vi "gui_T1.vi"(10 "input_xyz":T1) -> ()   [LabVIEW 2018]
uses:
  <vilib>/Analysis/NI_AALBase.lvlib
panel:
  out "particle_lost":bool
  in  "recenter_period_s":u32=5
  in  "recenter":bool=TRUE
  in  "show_all":bool
  in  "hide_all":bool
  out "elapsed_time_HMS":string
  out "estimated_time_HMS":string
  in  "plot_pulses":bool
  in  "gates_calculation":enum16{"Software", "Hardware"}(ring)=enum."Hardware"
  out "pulses":u32[][](graph)
  out "detections":u32[](graph)
  out "std. dev.":dbl format="%.3f"
  out "mean":dbl format="%0.2f"
  in  "auto_normalize":bool
  in  "normalize":bool
  in  "normalization_value":dbl=1.0 caption="Normalization value:" min=1.0 step=1.0
  out "status":string
  in  "use_proposed_width":bool
  in  "calc_width":bool
  in  "start":bool caption="Start"
  in  "save_file":bool
  out "contrast":dbl caption="Contrast :" format="%#_3f"
  in  "show_photons":bool
  in  "show_flags":bool
  out "mse":cluster{"read_widths_us":dbl[], "mse":dbl[]}(graph)
  in  "use_proposed_correction":bool
  out "proposed_read_width_us":dbl
  out "proposed_correction_us":dbl
  out "histogram":cluster{"histogram":i32[], "q_photons":i32[]}(graph)
  out "file_name":string caption="File name :"
  in  "sampling_mode":enum16{"Normal", "Sweep"}(ring)=enum."Sweep"
  out "quality":bool
  out "mse":dbl caption="Mean Square Error" format="%#.2e"
  out "T1_us":dbl format="%#.3g"
  out "T1 curves":cluster{dbl[], "dark_time_us":dbl[]}[](graph)
  in  "correction_us":dbl=0.65 caption="Delay"
  out "stop_count_photon":u32(colorbox)=16776704 caption="Stop Count & photon"
  out "stop_count":u32(colorbox)=6618880 caption="Stop Count"
  out "start_count_photon":u32(colorbox)=14417925 caption="Start Count & photon"
  out "start_count":u32(colorbox)=255 caption="Start Count"
  out "photon":u32(colorbox)=16448250 caption="Photon"
  out "noPhoton":u32(colorbox) caption="No Photon"
  out "photons_chart":u32[][](graph)
  in  "load_file":bool
  in  "refit":bool
  in  "read_width_us":dbl=1.0 caption="Width" min=0.0 max=10000.0 format="%#.3f"
  in  "read_delay_us":dbl caption="Delay"
  out "min_step":dbl format="%#.3f"
  in  "q_samples":i32=50
  in  "dt_stop_us":dbl=10000.0
  in  "dt_start_us":dbl=0.2
  in  "stop":bool
  in  "repetitions":i32=10000 caption="Repetitions" min=1 step=1
  in  "pulse_width_us":dbl=5.0 caption="Pulse width"
  # "Dark time [us]"
  # "*"
  # "*"
  # "us"
  # "*read_width_us and correction_us have to be multiple of 10ns\n*** start and stop markers are inside the detection gate. [start, stop]"
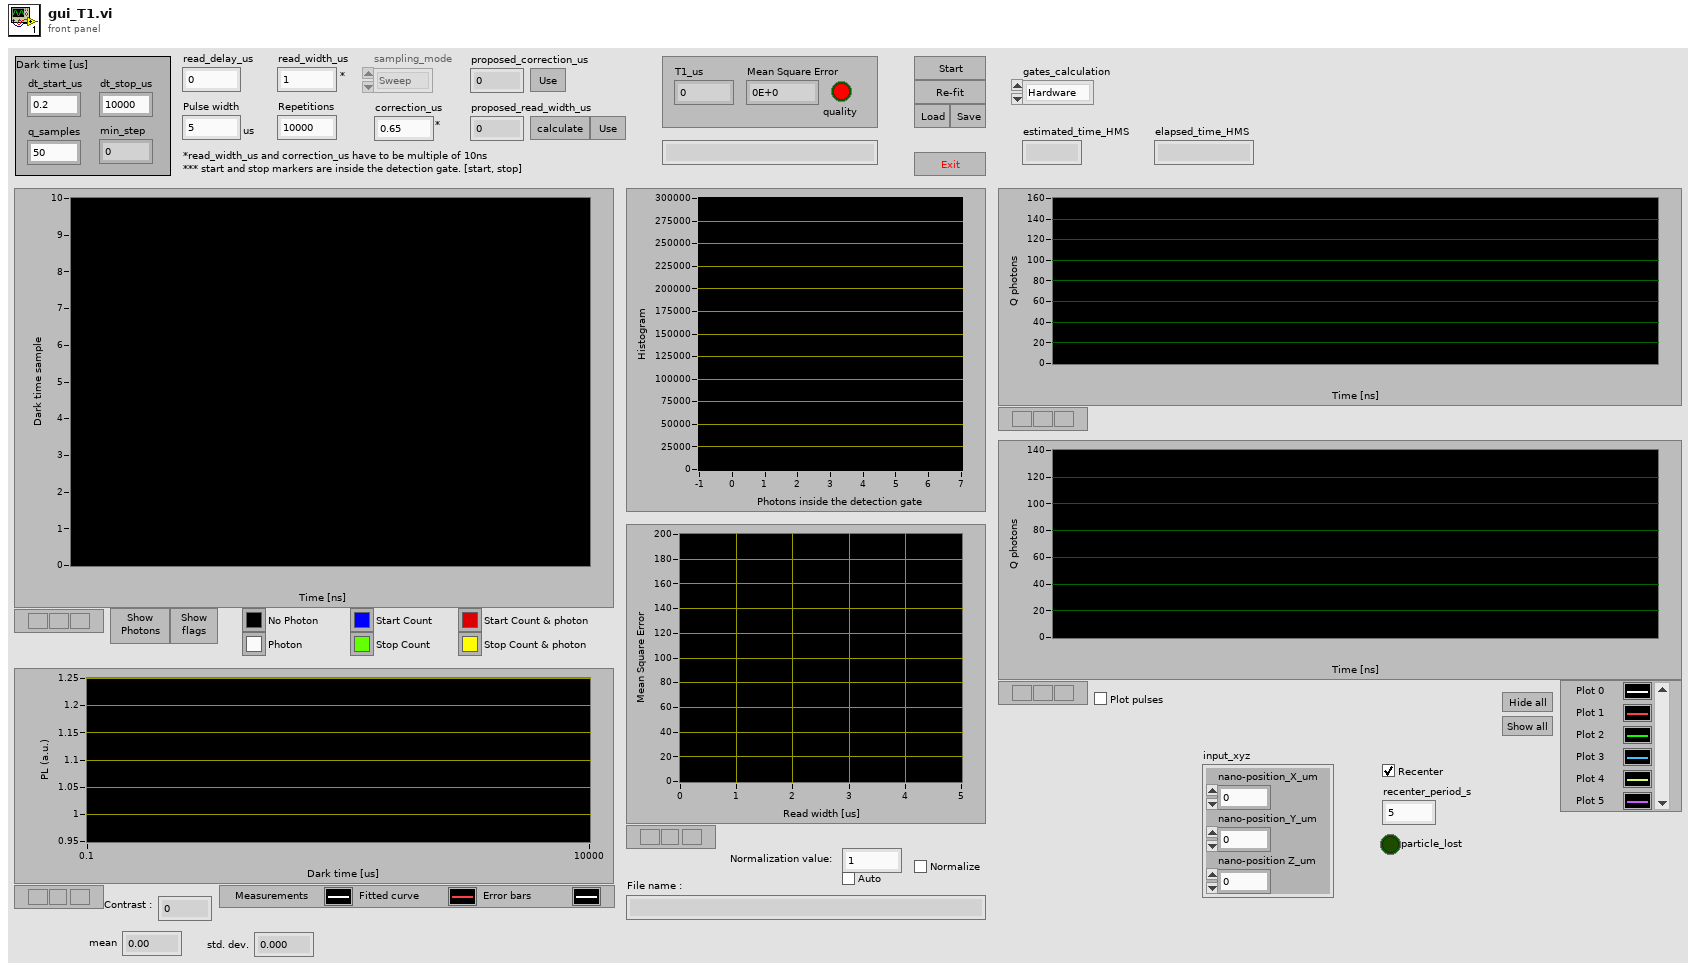
[diagram p1: front panel]
types:
  T1 = cluster{"nano-position_X_um":sgl, "nano-position_Y_um":sgl, "nano-position Z_um":sgl}
  T2 = cluster{"file_path":path, "file_name":string, "image":dbl[][][], "image_size_xy":cluster{"image_size_x_um":sgl, "image_size_y_um":sgl}, "pixel_dwell_time_ms":sgl, "Laser_power_mW":sgl, "pixel_size":dbl, "tile_ij":cluster{"tile_i":i32, "tile_j":i32}, "Objective":string, "ColorMarkers":cluster{dbl, u32}[], "timestamp":timestamp, "micro-position-xyz":cluster{"micro-position_x_mm":sgl, "micro-position_y_mm":sgl, "micro-position_z_mm":sgl}, "zero_xyz":cluster{"zero_x_mm":dbl, "zero_y_mm":dbl, "zero_z_mm":dbl}, "nano-position-xyz":cluster{"nano-position_x_V":sgl, "nano-position_y_V":sgl, "nano-position_z_V":sgl}, "Kxyz":cluster{"Kx_V/um":sgl, "Ky_V/um":sgl, "Kz_V/um":sgl}}
  T3 = cluster{"x_um":sgl[], "y_um":sgl[], "z_um":sgl[], "timetag":timestamp[]}
  T4 = cluster{"sampling_times":dbl[], "fitted_signal":dbl[]}
  T5 = cluster{"Ie":dbl, "Cm":dbl, "Tm":dbl, "C1":dbl, "T1":dbl, "mse":dbl}
  T6 = cluster{"dark_times_us":dbl[], "pulse_width_us":dbl, "read_delay_us":dbl, "read_width_us":dbl, "repetitions":i32, "sampling_mode":enum16{"Normal", "Sweep"}, "correction_us":dbl}
  T7 = cluster{"input_xyz":cluster{"nano-position_X_um":sgl, "nano-position_Y_um":sgl, "nano-position Z_um":sgl}, "recenter":bool, "recenter_s":u32}
  T8 = enum16{"standby", "doT1", "abort", "save", "re-fit", "load", "refresh", "use_proposed", "calcWidth"}
  T9 = cluster{"Ie":dbl, "A":dbl, "Ta":dbl, "B":dbl, "Tb":dbl, "mse":dbl}
  T10 = cluster{"dark_times":dbl[], "fitted_signal":dbl[]}
  T11 = cluster{"dark_times_us":dbl[], "measured_signal":dbl[]}
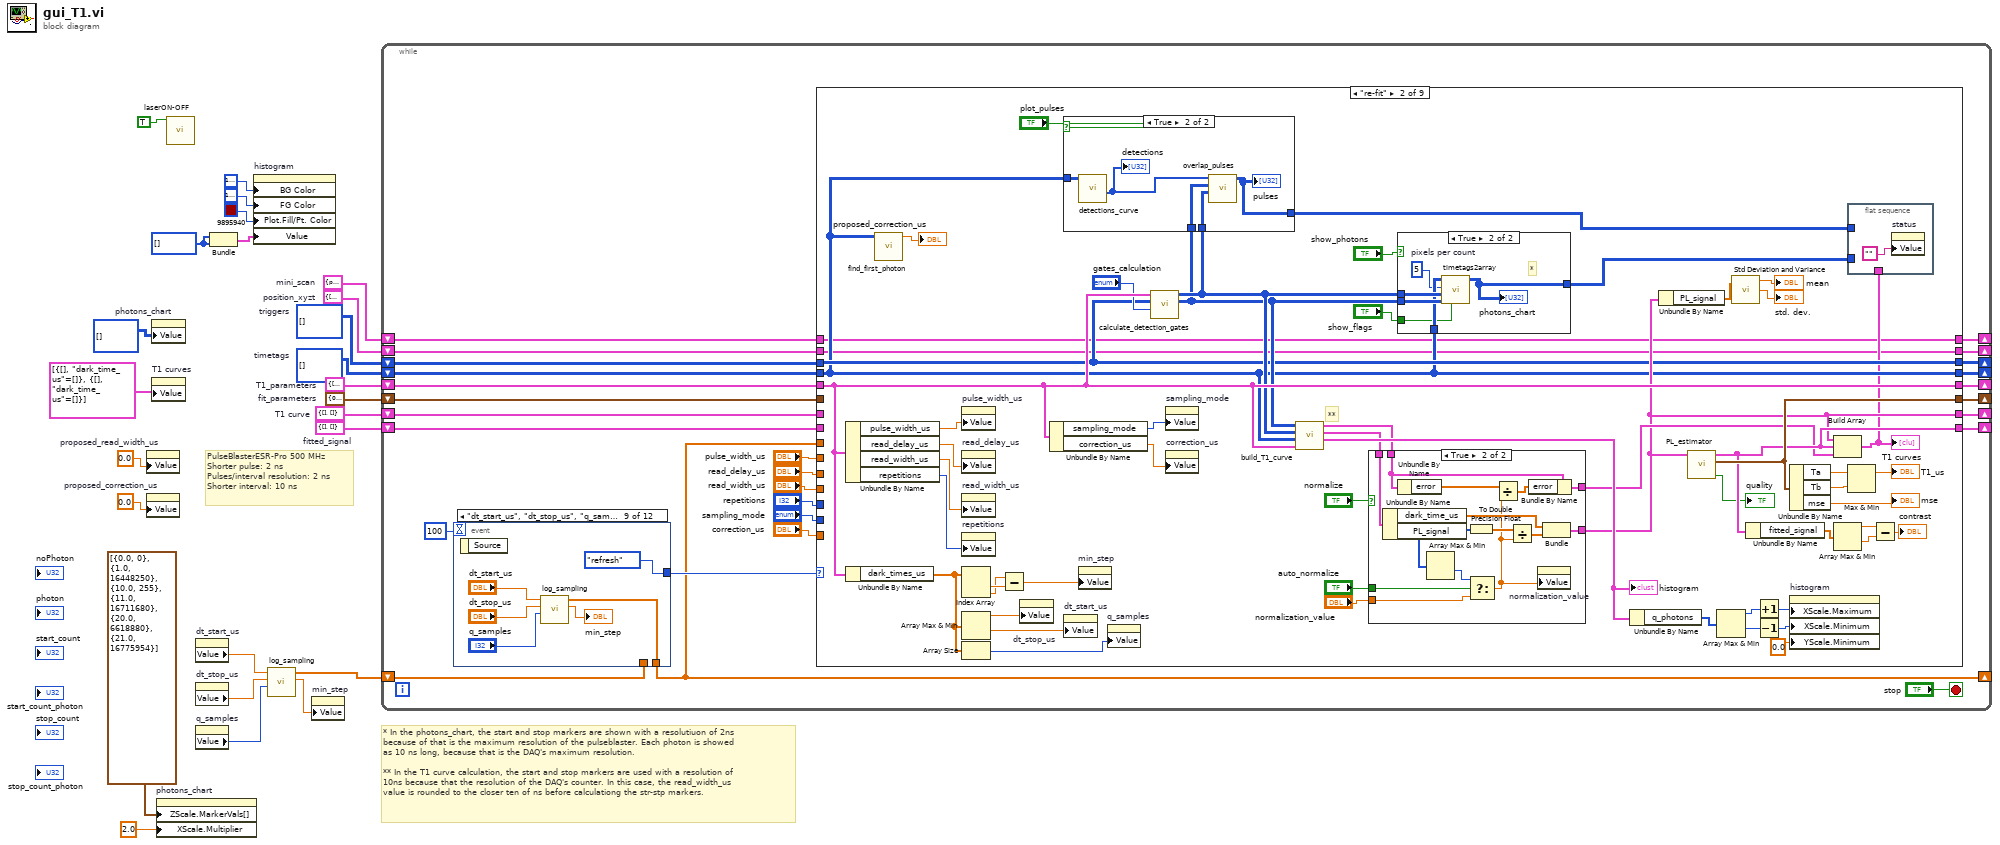
[diagram p0: block diagram]
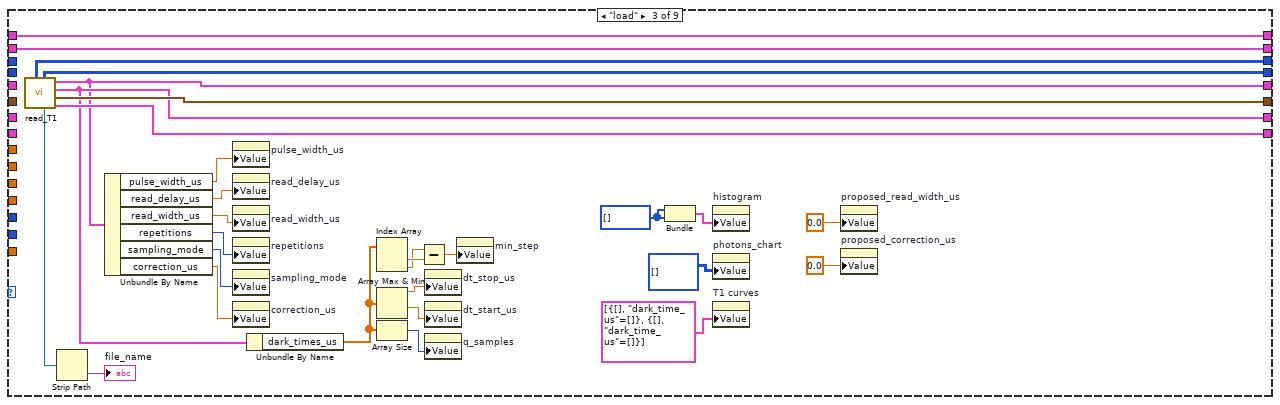
[diagram p6: hidden frame]
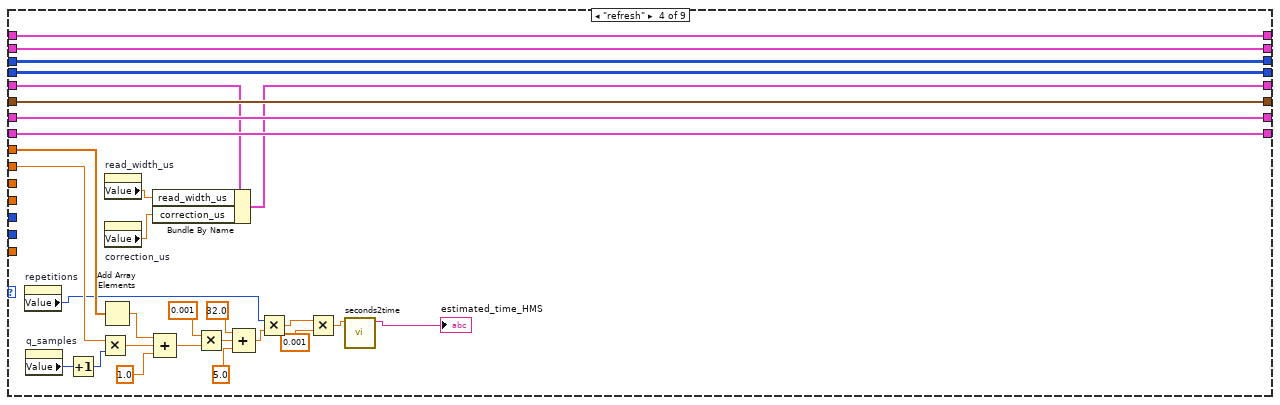
[diagram p7: hidden frame]
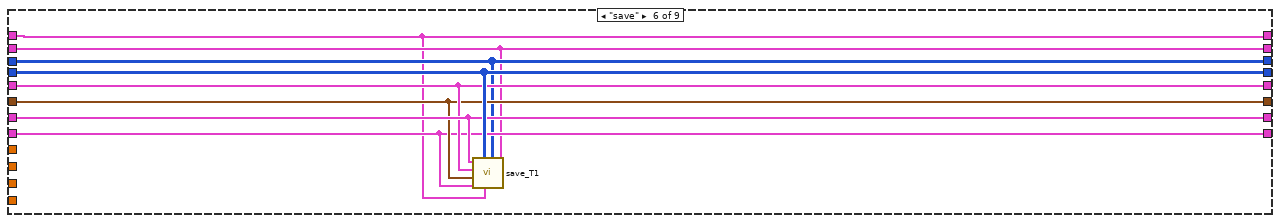
[diagram p9: hidden frame]
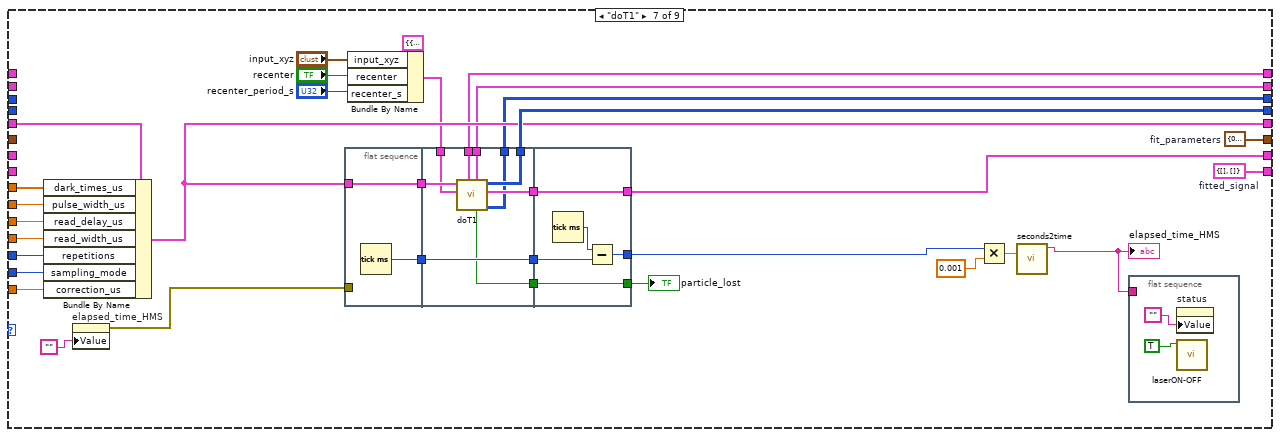
[diagram p10: hidden frame]
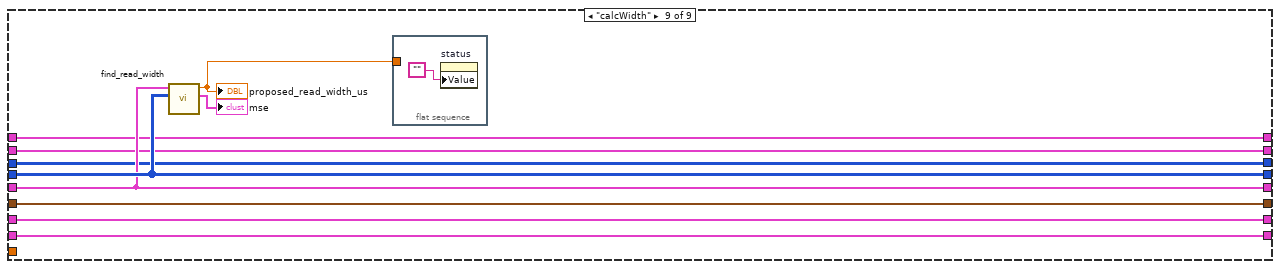
[diagram p12: hidden frame]
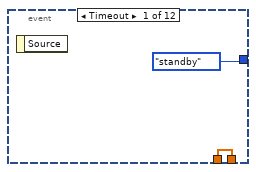
[diagram p13: hidden frame]
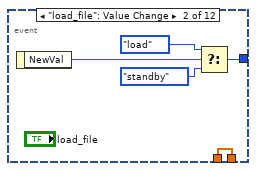
[diagram p14: hidden frame]
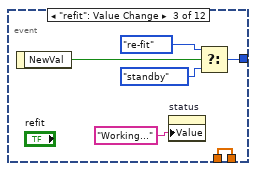
[diagram p15: hidden frame]
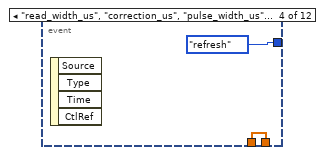
[diagram p16: hidden frame]
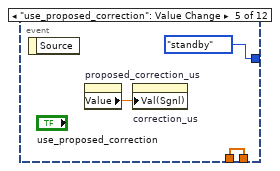
[diagram p17: hidden frame]
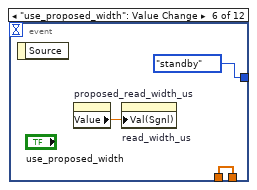
[diagram p18: hidden frame]
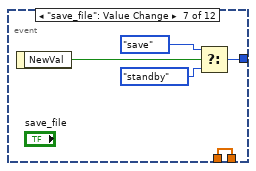
[diagram p19: hidden frame]
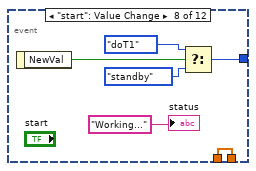
[diagram p20: hidden frame]
diagram:
  w1 = T2 {"file_path"=path "", "file_name"="", "image"=[], "image_size_xy"={"image_size_x_um"=0.0, "image_size_y_um"=0.0}, "pixel_dwell_time_ms"=0.0, "Laser_power_mW"=0.0, "pixel_size"=0.0, "tile_ij"={"tile_i"=0, "tile_j"=0}, "Objective"="", "ColorMarkers"=[], "timestamp"=timestamp(0 s since 1904-01-01), "micro-position-xyz"={"micro-position_x_mm"=0.0, "micro-position_y_mm"=0.0, "micro-position_z_mm"=0.0}, "zero_xyz"={"zero_x_mm"=0.0, "zero_y_mm"=0.0, "zero_z_mm"=0.0}, "nano-position-xyz"={"nano-position_x_V"=0.0, "nano-position_y_V"=0.0, "nano-position_z_V"=0.0}, "Kxyz"={"Kx_V/um"=0.0, "Ky_V/um"=0.0, "Kz_V/um"=0.0}}  # mini_scan
  w2 = T3 {"x_um"=[], "y_um"=[], "z_um"=[], "timetag"=[]}  # position_xyzt
  w4 = u32[][] []  # triggers
  w22 = T4 {"sampling_times"=[], "fitted_signal"=[]}  # fitted_signal
  w5 = u32[][] []  # timetags
  w23 = cluster{dbl[], "dark_time_us":dbl[]} {[], "dark_time_us"=[]}  # T1 curve
  w24 = T5 {"Ie"=0.0, "Cm"=0.0, "Tm"=0.0, "C1"=0.0, "T1"=0.0, "mse"=0.0}  # fit_parameters
  w21 = T6 {"dark_times_us"=[], "pulse_width_us"=0.0, "read_delay_us"=0.0, "read_width_us"=0.0, "repetitions"=0, "sampling_mode"=enum."Normal", "correction_us"=0.0}  # T1_parameters
  w16 = i32[] []
  # "* In the photons_chart, the start and stop markers are shown with a resolutiuon of 2ns \nbecause of that is the maximum resolution of the pulseblaster. Each photon is showed\nas 10 ns long, because that is the DAQ's maximum resolution.\n\n** In the T1 curve calculation, the start and stop markers are used with a resolution of\n10ns because that the resolution of the DAQ's counter. In this case, the read_width_us\nvalue is rounded to the closer ten of ns before calculationg the str-stp markers."
  # "PulseBlasterESR-Pro 500 MHz \nShorter pulse: 2 ns\nPulses/interval resolution: 2 ns\nShorter interval: 10 ns"
  n1 = property on="proposed_read_width_us" class="DigNum (strict)"("Value"=0.0 ("proposed_read_width_us")) -> ()  [unwired: 2 in, 2 out]
  n2 = property on="proposed_correction_us" class="DigNum (strict)"("Value"=0.0 ("proposed_correction_us")) -> ()  [unwired: 2 in, 2 out]
  n3 = property on="photons_chart" class="IntGraph (strict)"("Value"=i32[][] []) -> ()  [unwired: 2 in, 2 out]
  n4 = property on="T1 curves" class="XYGraph (strict)"("Value"=cluster{dbl[], "dark_time_us":dbl[]}[] [{[], "dark_time_us"=[]}, {[], "dark_time_us"=[]}] ("T1 curves")) -> ()  [unwired: 2 in, 2 out]
  n5 = property on="photons_chart" class="IntGraph (strict)"("ZScale.MarkerVals[]"=cluster{dbl, u32}[] [{0.0, 0}, {1.0, 16448250}, {10.0, 255}, {11.0, 16711680}, {20.0, 6618880}, {21.0, 16775954}] ("Z Scale.Marker Values[]"), "XScale.Multiplier"=2.0 ("X Scale.Offset and Multiplier:Multiplier")) -> ()  [unwired: 2 in, 2 out]
  n6 = call "laserON-OFF.vi"("ON-OFF"=TRUE) -> ()  [unwired: 10 in, 1 out]
  n7 = property on="dt_start_us" class="DigNum (strict)"() -> ("Value"=w8:dbl)  [unwired: 2 in, 2 out]
  n8 = property on="dt_stop_us" class="DigNum (strict)"() -> ("Value"=w9:dbl)  [unwired: 2 in, 2 out]
  n9 = property on="q_samples" class="DigNum (strict)"() -> ("Value"=w10:i32)  [unwired: 2 in, 2 out]
  n10 = Bundle(w16, w16) -> (w15:cluster{i32[], i32[]})  [unwired: 1 in]
  n11 = property on="histogram" class="XYGraph (strict)"("BG Color"=u32 16777222 ("Plot Area:Colors:FG Color"), "FG Color"=u32 16777228 ("Plot Area:Colors:FG Color"), "Plot.Fill/Pt. Color"=u32 9895940 ("Plot Area:Colors:FG Color"), "Value"=w15) -> ()  [unwired: 2 in, 2 out]
  n12 = call "log_sampling.vi"("q_samples"=w10, "stop_us"=w9, "start_us"=w8) -> ("min_step_us"=w11:dbl, "sampling_times_us"=w7:dbl[])  [unwired: 7 in]
  n13 = property on="min_step" class="DigNum (strict)"("Value"=w11) -> ()  [unwired: 2 in, 2 out]
  n14 = while {
    shift-right: [w42] -> _
    shift-left: w21 -> [w49]
    shift-right: [w41] -> _
    shift-left: w24 -> [w48]
    shift-right: [w40] -> _
    shift-left: w23 -> [w47]
    shift-right: [w46] -> _
    shift-left: w22 -> [w45]
    shift-right: [w43] -> _
    shift-left: w5 -> [w44]
    shift-right: [w32] -> _
    shift-left: w7 -> [w33]
    shift-right: [w31] -> _
    shift-left: w4 -> [w30]
    shift-right: [w29] -> _
    shift-left: w2 -> [w28]
    shift-right: [w26] -> _
    shift-left: w1 -> [w27]
    stop <- "stop" stop-if-true
    n15 = event shown="[8] \"dt_start_us\", \"dt_stop_us\", \"q_samples\": Value Change" {
      selector: _ -> [_ _ _ _ _ _ _ _ _ _ _ _]
      dyn-events: _ -> [_ _ _ _ _ _ _ _ _ _ _ _]
      timeout: 100 -> [_ _ _ _ _ _ _ _ _ _ _ _]
      tunnel: [T8."standby" w294 w300 T8."refresh" T8."standby" T8."standby" w313 w320 T8."refresh" w332 T8."standby" T8."standby"] -> w50
      tunnel: w33 -> [w289 w291 w297 w302 w304 w307 w310 w315 _ w328 w335 w341]
      tunnel: [w289 w291 w297 w302 w304 w307 w310 w315 w322 w328 w335 w341] -> w32
      event Timeout {
        n16 = event-data() -> ()  [unwired: 1 in, 1 out]
      }
      event "load_file": Value Change {
        n17 = event-data() -> ("NewVal"=w295:bool)  [unwired: 1 in]
        n18 = Select(t=T8."load", s=w295, f=T8."standby") -> (s? t:f=w294:T8)
      }
      event "refit": Value Change {
        n19 = event-data() -> ("NewVal"=w301:bool)  [unwired: 1 in]
        n20 = property on="status" class="Str"("Value"="Working...") -> ()  [unwired: 2 in, 2 out]
        n21 = Select(t=T8."re-fit", s=w301, f=T8."standby") -> (s? t:f=w300:T8)
      }
      event "read_width_us", "correction_us", "pulse_width_us", "repetitions": Value Change {
        n22 = event-data() -> ()  [unwired: 1 in, 4 out]
      }
      event "use_proposed_correction": Value Change {
        n23 = event-data() -> ()  [unwired: 1 in, 1 out]
        n24 = property on="proposed_correction_us" class="DigNum (strict)"() -> ("Value"=w306:dbl)  [unwired: 2 in, 2 out]
        n25 = property on="correction_us" class="DigNum (strict)"("Val(Sgnl)"=w306) -> ()  [unwired: 2 in, 2 out]
      }
      event "use_proposed_width": Value Change {
        n26 = event-data() -> ()  [unwired: 1 in, 1 out]
        n27 = property on="proposed_read_width_us" class="DigNum (strict)"() -> ("Value"=w309:dbl)  [unwired: 2 in, 2 out]
        n28 = property on="read_width_us" class="DigNum (strict)"("Val(Sgnl)"=w309) -> ()  [unwired: 2 in, 2 out]
      }
      event "save_file": Value Change {
        n29 = event-data() -> ("NewVal"=w314:bool)  [unwired: 1 in]
        n30 = Select(t=T8."save", s=w314, f=T8."standby") -> (s? t:f=w313:T8)
      }
      event "start": Value Change {
        n31 = event-data() -> ("NewVal"=w319:bool)  [unwired: 1 in]
        n32 = Select(t=T8."doT1", s=w319, f=T8."standby") -> (s? t:f=w320:T8)
        "status" <- "Working..."
      }
      event "dt_start_us", "dt_stop_us", "q_samples": Value Change {
        n33 = event-data() -> ()  [unwired: 1 in, 1 out]
        n34 = call "log_sampling.vi"("q_samples"="q_samples", "stop_us"="dt_stop_us", "start_us"="dt_start_us") -> ("min_step_us"=→"min_step":dbl, "sampling_times_us"=w322:dbl[])  [unwired: 7 in]
      }
      event "calc_width": Value Change {
        n35 = event-data() -> ("NewVal"=w331:bool)  [unwired: 1 in]
        n36 = property on="status" class="Str"("Value"="Working...") -> ()  [unwired: 2 in, 2 out]
        n37 = Select(t=T8."calcWidth", s=w331, f=T8."standby") -> (s? t:f=w332:T8)
      }
      event "hide_all": Value Change {
        n38 = event-data() -> ()  [unwired: 1 in, 1 out]
        n39 = property on="q_samples" class="DigNum (strict)"() -> ("Value"=w333:i32)  [unwired: 2 in, 2 out]
        n40 = Increment(x=w333) -> (x+1=w334:i32)
        n41 = for {
          N: w334 -> [_]
          i -> [w338]
          n42 = property on="pulses" class="WFGraph (strict)"("Active Plot"=w338, "Plot.Visible?"=FALSE ("Plot.Visible")) -> ()  [unwired: 2 in, 2 out]
        }
      }
      event "show_all": Value Change {
        n43 = event-data() -> ()  [unwired: 1 in, 1 out]
        n44 = property on="q_samples" class="DigNum (strict)"() -> ("Value"=w339:i32)  [unwired: 2 in, 2 out]
        n45 = Increment(x=w339) -> (x+1=w340:i32)
        n46 = for {
          N: w340 -> [_]
          i -> [w344]
          n47 = property on="pulses" class="WFGraph (strict)"("Active Plot"=w344, "Plot.Visible?"=TRUE ("Plot.Visible")) -> ()  [unwired: 2 in, 2 out]
        }
      }
    }
    n48 = case shown="\"re-fit\"" w50 {
      tunnel: w49 -> [w60 w94 _ w198 w209 w216 w251 w276 w285]
      tunnel: w48 -> [w59 _ _ w201 w208 w215 _ w275 w284]
      tunnel: w47 -> [w58 _ _ w200 w207 w217 _ w274 w283]
      tunnel: [w57 w91 w173 w199 w206 w214 w231 w273 w282] -> w46
      tunnel: w45 -> [w57 _ _ w199 w206 w214 _ w273 w282]
      tunnel: [w56 w69 w164 w202 w210 w218 w250 w277 w286] -> w43
      tunnel: w44 -> [w56 w69 _ w202 w210 w218 _ w277 w286]
      tunnel: [w60 w94 w166 w197 w209 w216 w241 w276 w285] -> w42
      tunnel: [w59 w116 w172 w201 w208 w215 w230 w275 w284] -> w41
      tunnel: [w58 w79 w171 w200 w207 w217 w242 w274 w283] -> w40
      tunnel: "read_delay_us" -> [_ _ _ _ _ _ w249 _ _]
      tunnel: "pulse_width_us" -> [_ _ _ w192 _ _ w248 _ _]
      tunnel: "read_width_us" -> [_ _ _ _ _ _ w247 _ _]
      tunnel: "repetitions" -> [_ _ _ _ _ _ w246 _ _]
      tunnel: "sampling_mode" -> [_ _ _ _ _ _ w245 _ _]
      tunnel: "correction_us" -> [_ _ _ _ _ _ w244 _ _]
      tunnel: w32 -> [_ _ _ w193 _ _ w243 _ _]
      tunnel: [w55 w70 w147 w194 w205 w213 w240 w272 w280] -> w31
      tunnel: w30 -> [w55 w70 _ w194 w205 w213 _ w272 w280]
      tunnel: [w54 w65 w146 w175 w204 w212 w224 w271 w279] -> w29
      tunnel: w28 -> [w54 w65 w146 w175 w204 w212 _ w271 w279]
      tunnel: [w53 w64 w145 w174 w203 w211 w221 w270 w278] -> w26
      tunnel: w27 -> [w53 w64 w145 w174 w203 w211 _ w270 w278]
      frame "standby", Default {
      }
      frame "re-fit" {
        # "**"
        n49 = Unbundle By Name(w94) -> ("pulse_width_us"=w108:dbl, "read_delay_us"=w107:dbl, "read_width_us"=w106:dbl, "repetitions"=w105:i32)
        n50 = Unbundle By Name(w94) -> ("dark_times_us"=w113:dbl[])
        n51 = call "find_first_photon.vi"("timetags"=w69) -> ("Numeric"=→"proposed_correction_us":dbl)  [unwired: 10 in]
        n52 = property on="pulse_width_us" class="DigNum (strict)"("Value"=w108) -> ()  [unwired: 2 in, 2 out]
        n53 = property on="read_delay_us" class="DigNum (strict)"("Value"=w107) -> ()  [unwired: 2 in, 2 out]
        n54 = property on="read_width_us" class="DigNum (strict)"("Value"=w106) -> ()  [unwired: 2 in, 2 out]
        n55 = property on="repetitions" class="DigNum (strict)"("Value"=w105) -> ()  [unwired: 2 in, 2 out]
        n56 = Index Array(array=w113) -> (element #1=w115:dbl, element #2=w114:dbl)  [unwired: 2 in]
        n57 = Array Max & Min(array=w113) -> (max value=w112:dbl, min value=w111:dbl)  [unwired: 2 out]
        n58 = Array Size(array=w113) -> (size(s)=w110:i32)
        n59 = Subtract(x=w114, y=w115) -> (x-y=w109:dbl)
        n60 = property on="dt_stop_us" class="DigNum (strict)"("Value"=w112) -> ()  [unwired: 2 in, 2 out]
        n61 = Unbundle By Name(w94) -> ("sampling_mode"=w104:enum16{"Normal", "Sweep"}, "correction_us"=w103:dbl)
        n62 = property on="dt_start_us" class="DigNum (strict)"("Value"=w111) -> ()  [unwired: 2 in, 2 out]
        n63 = property on="min_step" class="DigNum (strict)"("Value"=w109) -> ()  [unwired: 2 in, 2 out]
        n64 = property on="q_samples" class="DigNum (strict)"("Value"=w110) -> ()  [unwired: 2 in, 2 out]
        n65 = call "calculate_detection_gates.vi"("gates_calculation"="gates_calculation", "triggers"=w70, "T1_parameters"=w94) -> ("start_read"=w74:u32[][], "stop_read"=w75:u32[][])  [unwired: 7 in]
        n66 = case shown="True" "plot_pulses" {
          tunnel: w75 -> [_ w122]
          tunnel: w74 -> [_ w121]
          tunnel: w69 -> [_ w120]
          tunnel: [_ w118] -> w66
          frame False {
          }
          frame True {
            n67 = call "detections_curve.vi"("timetags"=w120) -> ("detections"=w119:u32[])  [unwired: 10 in]
            "detections" <- w119
            n68 = call "overlap_pulses.vi"("stop_read"=w122, "start_read"=w121, "detections"=w119) -> ("pulses"=w118:u32[][])  [unwired: 8 in]
            "pulses" <- w118
          }
        }
        n69 = property on="sampling_mode" class="Enum (strict)"("Value"=w104) -> ()  [unwired: 2 in, 2 out]
        n70 = property on="correction_us" class="DigNum (strict)"("Value"=w103) -> ()  [unwired: 2 in, 2 out]
        n71 = call "build_T1_curve.vi"("T1_parameters"=w94, "timetags"=w69, "stop_read"=w75, "start_read"=w74) -> ("histogram"=w102:cluster{"q_photons":i32[], "histogram":i32[]}, "T1 curve"=w73:cluster{"dark_time_us":dbl[], "PL_signal":i32[]}, "error_bars"=w82:cluster{"dark_times_us":dbl[], "error":dbl[]})  [unwired: 5 in]
        "histogram" <- w102
        n72 = case shown="True" "normalize" {
          tunnel: [w123 w138] -> w79
          tunnel: "normalization_value" -> [_ w129]
          tunnel: w82 -> [w124 w133]
          tunnel: [w124 w131] -> w81
          tunnel: "auto_normalize" -> [_ w127]
          tunnel: w73 -> [w123 w125]
          frame False {
          }
          frame True {
            n73 = Unbundle By Name(w125) -> ("dark_time_us"=w136:dbl[], "PL_signal"=w130:i32[])
            n74 = Unbundle By Name(w133) -> ("error"=w134:dbl[])
            n75 = Array Max & Min(array=w130) -> (min value=w128:i32)  [unwired: 3 out]
            n76 = To Double Precision Float(number=w130) -> (double precision float=w135:dbl[])
            n77 = Select(t=w128, s=w127, f=w129) -> (s? t:f=w126:dbl)
            n78 = Divide(x=w134, y=w126) -> (x/y=w132:dbl[])
            n79 = Divide(x=w135, y=w126) -> (x/y=w137:dbl[])
            n80 = Bundle By Name(cluster=w133, "error"=w132) -> (w131:cluster{"dark_times_us":dbl[], "error":dbl[]})
            n81 = property on="normalization_value" class="DigNum (strict)"("Value"=w126) -> ()  [unwired: 2 in, 2 out]
            n82 = Bundle("dark_time_us"=w136, w137) -> (w138:cluster{"dark_time_us":dbl[], dbl[]})  [unwired: 1 in]
          }
        }
        n83 = case shown="True" "show_photons" {
          tunnel: w74 -> [_ w144]
          tunnel: w75 -> [_ w143]
          tunnel: w69 -> [_ w142]
          tunnel: "show_flags" -> [_ w141]
          tunnel: [_ w139] -> w67
          frame False {
          }
          frame True {
            w140 = u32 5  # pixels per count
            # "*"
            n84 = call "timetags2array.vi"("show_flags"=w141, "start_read"=w144, "stop_read"=w143, "pixels/count"=w140, "timetags"=w142) -> ("photons_chart"=w139:u32[][])  [unwired: 6 in]
            "photons_chart" <- w139
          }
        }
        n85 = Unbundle By Name(w102) -> ("q_photons"=w101:i32[])
        n86 = Unbundle By Name(w79) -> ("PL_signal"=w78:dbl[])
        n87 = call "PL_estimator.vi"("measured_signal"=w79) -> ("quality_check"=→"quality":bool, "fit_parameters"=w116:T9, "fitted_signal"=w91:T4)  [unwired: 8 in]
        n88 = Array Max & Min(array=w101) -> (max value=w100:i32, min value=w98:i32)  [unwired: 2 out]
        n89 = call <vilib>:"Std Deviation and Variance.vi"("X"=w78) -> ("mean"=→"mean":dbl, "standard deviation"=→"std. dev.":dbl)  [unwired: 1 in, 1 out]
        n90 = Unbundle By Name(w91) -> ("fitted_signal"=w90:dbl[])
        n91 = Increment(x=w100) -> (x+1=w99:i32)
        n92 = Decrement(x=w98) -> (x-1=w97:i32)
        n93 = Unbundle By Name(w116) -> ("Ta"=w63:dbl, "Tb"=w62:dbl, "mse"=→"mse":dbl)
        n94 = property on="histogram" class="XYGraph (strict)"("XScale.Maximum"=w99, "XScale.Minimum"=w97, "YScale.Minimum"=0.0 ("Y Scale.Range:Minimum")) -> ()  [unwired: 2 in, 2 out]
        n95 = Build Array(w79, w91, w81) -> (w68:cluster{"dark_times_us":dbl[], "error":dbl[]}[])
        "T1 curves" <- w68
        n96 = Array Max & Min(array=w90) -> (max value=w89:dbl, min value=w88:dbl)  [unwired: 2 out]
        n97 = flat-sequence {
          tunnel: w68 -> [_]
          tunnel: w67 -> [_]
          tunnel: w66 -> [_]
          frame #0 {
            n98 = property on="status" class="Str"("Value"="") -> ()  [unwired: 2 in, 2 out]
          }
        }
        n99 = Max & Min(x=w63, y=w62) -> (max(x,y)=→"T1_us":dbl)  [unwired: 1 out]
        n100 = Subtract(x=w89, y=w88) -> (x-y=→"contrast":dbl)
      }
      frame "load" {
        w161 = i32[] []
        n101 = call "read_T1.vi"() -> ("fitted_signal"=w173:T10, "fit_parameters"=w172:T5, "T1_curve"=w171:T11, "T1_parameters"=w166:T6, "file_path"=w163:path, "timetags"=w164:u32[][], "triggers"=w147:u32[][])  [unwired: 5 in]
        n102 = Strip Path(path=w163) -> (name=→"file_name":string)  [unwired: 1 out]
        n103 = Unbundle By Name(w166) -> ("pulse_width_us"=w155:dbl, "read_delay_us"=w154:dbl, "read_width_us"=w167:dbl, "repetitions"=w152:i32, "sampling_mode"=w153:enum16{"Normal", "Sweep"}, "correction_us"=w165:dbl)
        n104 = property on="pulse_width_us" class="DigNum (strict)"("Value"=w155) -> ()  [unwired: 2 in, 2 out]
        n105 = property on="read_delay_us" class="DigNum (strict)"("Value"=w154) -> ()  [unwired: 2 in, 2 out]
        n106 = property on="read_width_us" class="DigNum (strict)"("Value"=w167) -> ()  [unwired: 2 in, 2 out]
        n107 = property on="repetitions" class="DigNum (strict)"("Value"=w152) -> ()  [unwired: 2 in, 2 out]
        n108 = property on="sampling_mode" class="Enum (strict)"("Value"=w153) -> ()  [unwired: 2 in, 2 out]
        n109 = property on="correction_us" class="DigNum (strict)"("Value"=w165) -> ()  [unwired: 2 in, 2 out]
        n110 = Unbundle By Name(w171) -> ("dark_times_us"=w170:dbl[])
        n111 = Index Array(array=w170) -> (element #1=w169:dbl, element #2=w168:dbl)  [unwired: 2 in]
        n112 = Array Max & Min(array=w170) -> (max value=w149:dbl, min value=w150:dbl)  [unwired: 2 out]
        n113 = Array Size(array=w170) -> (size(s)=w151:i32)
        n114 = Subtract(x=w168, y=w169) -> (x-y=w148:dbl)
        n115 = property on="dt_stop_us" class="DigNum (strict)"("Value"=w149) -> ()  [unwired: 2 in, 2 out]
        n116 = property on="dt_start_us" class="DigNum (strict)"("Value"=w150) -> ()  [unwired: 2 in, 2 out]
        n117 = property on="q_samples" class="DigNum (strict)"("Value"=w151) -> ()  [unwired: 2 in, 2 out]
        n118 = property on="min_step" class="DigNum (strict)"("Value"=w148) -> ()  [unwired: 2 in, 2 out]
        n119 = Bundle(w161, w161) -> (w160:cluster{i32[], i32[]})  [unwired: 1 in]
        n120 = property on="histogram" class="XYGraph (strict)"("Value"=w160) -> ()  [unwired: 2 in, 2 out]
        n121 = property on="photons_chart" class="IntGraph (strict)"("Value"=i32[][] []) -> ()  [unwired: 2 in, 2 out]
        n122 = property on="T1 curves" class="XYGraph (strict)"("Value"=cluster{dbl[], "dark_time_us":dbl[]}[] [{[], "dark_time_us"=[]}, {[], "dark_time_us"=[]}] ("T1 curves")) -> ()  [unwired: 2 in, 2 out]
        n123 = property on="proposed_read_width_us" class="DigNum (strict)"("Value"=0.0 ("proposed_read_width_us")) -> ()  [unwired: 2 in, 2 out]
        n124 = property on="proposed_correction_us" class="DigNum (strict)"("Value"=0.0 ("proposed_correction_us")) -> ()  [unwired: 2 in, 2 out]
      }
      frame "refresh" {
        n125 = property on="repetitions" class="DigNum (strict)"() -> ("Value"=w180:i32)  [unwired: 2 in, 2 out]
        n126 = property on="q_samples" class="DigNum (strict)"() -> ("Value"=w191:i32)  [unwired: 2 in, 2 out]
        n127 = Increment(x=w191) -> (x+1=w190:i32)
        n128 = Multiply(x=w192, y=w190) -> (x*y=w188:dbl)
        n129 = Add Array Elements(numeric array=w193) -> (sum=w189:dbl)
        n130 = property on="read_width_us" class="DigNum (strict)"() -> ("Value"=w196:dbl)  [unwired: 2 in, 2 out]
        n131 = property on="correction_us" class="DigNum (strict)"() -> ("Value"=w195:dbl)  [unwired: 2 in, 2 out]
        n132 = Bundle By Name(cluster=w198, "read_width_us"=w196, "correction_us"=w195) -> (w197:T6)
        n133 = Compound Arithmetic op=ADD(w189, w188, 1.0 ("value")) -> (w186:dbl)
        n134 = Multiply(x=0.001, y=w186) -> (x*y=w184:dbl)
        n135 = Compound Arithmetic op=ADD(32.0 ("value"), w184, 5.0 ("value")) -> (w181:dbl)
        n136 = Multiply(x=w180, y=w181) -> (x*y=w179:dbl)
        n137 = Multiply(x=w179, y=0.001 ("x")) -> (x*y=w177:dbl)
        n138 = call "seconds2time.vi"("seconds"=w177) -> ("HH:MM:SS"=→"estimated_time_HMS":string)  [unwired: 10 in]
      }
      frame "use_proposed" {
      }
      frame "save" {
        n139 = call "save_T1.vi"("position_xyzt"=w212, "triggers"=w213, "image_info"=w211, "timetags"=w218, "fitted_signal_in"=w214, "fit_parameters"=w215, "T1_parameters"=w216, "T1_curve_in"=w217) -> ()  [unwired: 4 in]
      }
      frame "doT1" {
        w230 = T5 {"Ie"=0.0, "Cm"=0.0, "Tm"=0.0, "C1"=0.0, "T1"=0.0, "mse"=0.0}  # fit_parameters
        w231 = T4 {"sampling_times"=[], "fitted_signal"=[]}  # fitted_signal
        n140 = Bundle By Name(cluster=w251, "dark_times_us"=w243, "pulse_width_us"=w248, "read_delay_us"=w249, "read_width_us"=w247, "repetitions"=w246, "sampling_mode"=w245, "correction_us"=w244) -> (w241:T6)
        n141 = property on="elapsed_time_HMS" class="Str"("Value"="") -> (error out=w233:errorcluster)  [unwired: 2 in, 1 out]
        n142 = flat-sequence {
          tunnel: w241 -> [w253]
          tunnel: [w253] -> w239
          tunnel: [w252] -> w236
          tunnel: w233 -> [_]
          tunnel: [w262] -> w250
          tunnel: [w259] -> w240
          tunnel: w239 -> [w260]
          tunnel: [w261] -> w238
          tunnel: [w258] -> w237
          tunnel: w236 -> [w258]
          tunnel: w227 -> [w257]
          tunnel: [w256] -> w224
          tunnel: [w255] -> w221
          tunnel: [w254] -> w220
          tunnel: [w267] -> w242
          tunnel: w238 -> [w267]
          tunnel: w237 -> [w265]
          tunnel: [w264] -> w228
          tunnel: w220 -> [w263]
          tunnel: [w263] -> w219
          frame #0 {
            n143 = Tick Count (ms)() -> (millisecond timer value=w252:u32)
          }
          frame #1 {
            n144 = call "doT1.vi"("parameters_recenter"=w257, "T1_parameters"=w260) -> ("triggers"=w259:u32[][], "T1 curve"=w261:cluster{dbl[], "dark_time_us":dbl[]}, "timetags"=w262:u32[][], "particle_lost"=w254:bool, "position_xyz"=w256:T3, "mini_scan"=w255:T2)  [unwired: 3 in, 1 out]
          }
          frame #2 {
            n145 = Tick Count (ms)() -> (millisecond timer value=w266:u32)
            n146 = Subtract(x=w266, y=w265) -> (x-y=w264:u32)
          }
        }
        n147 = Bundle By Name(cluster=T7 {"input_xyz"={"nano-position_X_um"=0.0, "nano-position_Y_um"=0.0, "nano-position Z_um"=0.0}, "recenter"=FALSE, "recenter_s"=3} ("parameters_recenter"), "input_xyz"="input_xyz", "recenter"="recenter", "recenter_s"="recenter_period_s") -> (w227:T7)
        n148 = Multiply(x=w228, y=0.001) -> (x*y=w235:dbl)
        n149 = call "seconds2time.vi"("seconds"=w235) -> ("HH:MM:SS"=w229:string)  [unwired: 10 in]
        "elapsed_time_HMS" <- w229
        n150 = flat-sequence {
          tunnel: w229 -> [_]
          frame #0 {
            n151 = property on="status" class="Str"("Value"="") -> ()  [unwired: 2 in, 2 out]
            n152 = call "laserON-OFF.vi"("ON-OFF"=TRUE) -> ()  [unwired: 10 in, 1 out]
          }
        }
        "particle_lost" <- w219
      }
      frame "abort" {
      }
      frame "calcWidth" {
        n153 = call "find_read_width.vi"("timetags"=w286, "T1_parameters"=w285) -> ("mse"=→"mse":cluster{"read_widths_us":dbl[], "mse":dbl[]}, "proposed_read_width_us"=w281:dbl)  [unwired: 8 in]
        "proposed_read_width_us" <- w281
        n154 = flat-sequence {
          tunnel: w281 -> [_]
          frame #0 {
            n155 = property on="status" class="Str"("Value"="") -> ()  [unwired: 2 in, 2 out]
          }
        }
      }
    }
  }
